vi "AlliGator Phasor Plot Image ROI Storage [MULT] v3.vi"(7 "Curent ROI Colors":u32[](array[colorbox]), 8 "Error In":errorcluster, 9 "Current ROI Descriptor(s)":T2[](array[typedef]) {"Contours"."Type" items=["No Selection", "Point", "Line", "Rectangle", "Oval", "Polygon", "Freehand Region", "Annulus", "Unused2", "Unused3", "Broken Line", "Freehand Line", "Rotated Rectangle"]}, 10 "Default Name(s) (\"ROI\")":string[](array[string]), 11 "Action":T1=enum."Update Current ROI Descriptor") -> (0 "Error Out":errorcluster, 1 "Current ROI Descriptors":T2[](array[typedef]) {"Contours"."Type" items=["No Selection", "Point", "Line", "Rectangle", "Oval", "Polygon", "Freehand Region", "Annulus", "Unused2", "Unused3", "Broken Line", "Freehand Line", "Rotated Rectangle"]}, 2 "Current ROI Names":string[](array[string]), 3 "Current Phasor Plot Image ROI":i32, 4 "Old ROI Name":string, 5 "Curent ROI Colors":u32[](array[colorbox]))   [LabVIEW 2021, in "AlliGator ROIs.lvlib"]
doc: "Handles multiple Phasor Plot image ROIs storage."
uses:
  AlliGator ROIs.lvlib
  AlliGator ROI Manager Actions.ctl
  Globals, Variables, Constants/AlliGator Variables List.ctl
  Image/Named ROI Description.ctl
  AlliGator Image ROI Event refnum.ctl
  Variant/Variant to Data/Variant to I32.vi
  <userlib>/_OpenG.lib/array/array.llb/Sort 1D Array (I32)__ogtk.vi
  Image/Image.lvlib
  Globals, Variables, Constants/AlliGator Globals, Variables & Constants.lvlib
  Variant/Variant to Data/Variant to Data.lvlib
  <userlib>/_OpenG.lib/array/array.llb/openg_array.lvlib
  Strings/Strings.lvlib
panel:
  # "see the AlliGator License on the block diagram (Ctrl+E or Window:Show Block Diagram)"
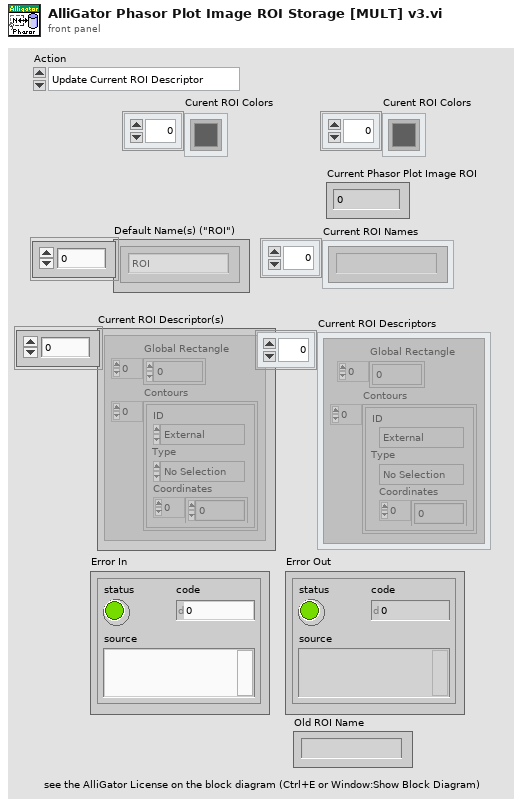
[diagram p1: front panel]
types:
  T1 = typedef "AlliGator ROIs.lvlib/AlliGator ROI Manager Actions.ctl" = enum16{"Undefined", "Delete Current ROI", "Delete All Unselected ROIs", "Delete Multiple ROIs", "Delete All ROIs", "Swap ROIs", "Insert ROI", "Update Current ROI Descriptor", "Rename Current ROI", "Store New ROI", "Store Multiple ROIs", "Select Next ROI", "Select Previous ROI", "Find Selected ROI", "Show All ROIs", "Update ROI Manager Window", "Merge All ROIs", "Unmerge ROI", "Set Selected ROI by ID"}
  T2 = typedef "ROI Descriptor" = cluster{"Global Rectangle":i32[], "Contours":cluster{"ID":enum32{"External", "Internal"}, "Type":u32, "Coordinates":i32[]}[]}
  T3 = typedef "AlliGator ROIs.lvlib/AlliGator Image ROI Event refnum.ctl" = refnum<user-event>
  T4 = typedef "AlliGator Globals, Variables & Constants.lvlib/AlliGator Variables List.ctl" = enum16{"---- GUI ----", "GUI:Initialization Status", "GUI:State Indicators Refnum", "GUI:Original AlliGator Menu Items", "GUI:Current Action Loop State", "GUI:Script in progress", "GUI:Playback", "GUI:Loop Playback", "GUI:Search ROI Used", "GUI:Search ROI", "Decay Graph Max Legend Size", "Intensity Graph Max Legend Size", "Decay Statistics Graph Max Legend Size", "Phasor Graph Max Legend Size", "Phasor Ratio Graph Max Legend Size", "Lifetime Graph Max Legend Size", "---- Files ----", "Files:Export Dataset Frames as Individual Files", "Files:Show Batch Export Help Balloons", "Files:Frames in Dataset", "Files:ptu File Frame Start Indices", "Files:Current Frame in Dataset", "Files:Current Frame Timestamp", "Files:Dataset Loaded", "Files:Dataset Metadata", "Files:Dataset Channel", "Files:Dataset Data Description", "Files:Background Dataset Metadata", "Files:Background Dataset Channel", "Files:Background Dataset Data Description", "Files:Background File Subtraction", "Files:Background File Path", "Files:Background File Pile-up Correction", "Files:Background File Pixel Well Capacity", "Files:Background File Scaling Factor", "Files:Current Dataset Load Settings", "Files:Dataset Path", "Files:ICCD-specific Information", "Files:Macrotime Gate Separation", "------ Python Plugins ------", "Python Plugins:Information", "Python Plugins:Python Session", "Python Plugins:Valid Python Session?", "---- Source Image ----", "Source Image:ROIs", "Source Image:Current ROI", "Source Image:ROI Event Refnum", "X_Source Image Display Range", "X_Source Image Palette Information", "X_Type of Displayed Image", "X_Time Gate Slider", "Source Image:Palette List", "Source Image:Scale", "Source Image:ROI Overlay Color", "Source Image:Overlay to Erase", "Source Image:Is Displayed Image Accumulated", "Source Image:White Light Image Modified", "Source Image:Mask Image Modified", "---- Image Profile Window ----", "Image Profile:Window Event Refnum", "Image Profile:IntensityType", "Image Profile:Intensity Average Type", "Image Profile:Intensity-weighted SDV", "Image Profile:Box Profile Type", "Image Profile:Window Open", "Image Profile:Plotted Fit Parameter", "------ Phasor Graph -------", "Phasor Graph:Show Line", "---- Phasor Plot ---", "Phasor Plot:Parameters Changed", "Phasor Plot:FLI Dataset Modified since last Calculation", "Phasor Harmonics Data", "Selected Phasor Harmonics", "Phasor Harmonic Manager Event Refnum", "Phasor Plot:ROIs", "Phasor Plot:Current ROI", "Phasor Plot:ROI Event Refnum", "Phasor Plot:Image Reference Points", "Phasor Plot:Computed", "Phasor Plot:Palette Information", "Phasor Plot:Palette List", "Phasor Plot:Phasor Ratio Palette Information", "Phasor Plot:Phasor Ratio Palette List", "Phasor Plot:Image Scale", "Phasor Plot:Image Overlay to Erase", "Phasor Plot:Image Elements to Update", "Phasor Plot:Current Calculation Parameters", "Phasor Plot:Current Calibration Options", "Phasor Plot:Reset Cumulated Phasor Plot", "Phasor Plot:Reference 1", "Phasor Plot:Lifetime Reference 1", "Phasor Plot:Reference 1 Frequency", "Phasor Plot:Reference 2", "Phasor Plot:Lifetime Reference 2", "Phasor Plot:Reference 2 Frequency", "---- Decay Analysis ----", "Number of Selected Decays to Fit", "LS Fit Results", "LAR Fit Results", "BS Fit Results", "Last Decay Max - Min", "Best Fit Parameters", "Best Fit Parameter Names", "Actual Size X", "Actual Size Y", "Binning X", "Binning Y", "Actual # Gates", "Dataset Number", "Gates to...", "Gates Skipped", "Gates to keep", "Gate Step", "Gate Separation", "Reversed Gates", "Pile-up Correction", "Pixel Well Capacity", "Background Subtracted", "Background Subtraction Method", "Background Definition Range", "Background File (deprecated)", "Number of Dataset Accumulated", "Array of Accumulated Dataset Paths", "Do Averaged Datasets", "Destination File Path", "Process Plot Target", "Use 1/D as Phasor Frequency", "---- Decay Fit Parameter Map -----", "Decay Fit Parameter Map:Palette Information", "Decay Fit Parameter Map:Palette List", "---- Parameter Map ----", "Parameter Map:Palette Information", "Parameter Map:Palette List", "------- Local Decay Window ---------", "Local Decay Graph Window:Event Refnum", "Local Decay Graph Window:Use normalized IRF for convolution", "----- Miscellaneous ----", "Misc:Skippable Dialog Windows Status"}
  T5 = typedef "Image.lvlib/Named ROI Description.ctl" = cluster{"ROI Descriptor":T2, "ROI Name":string, "Overlay Color":u32}
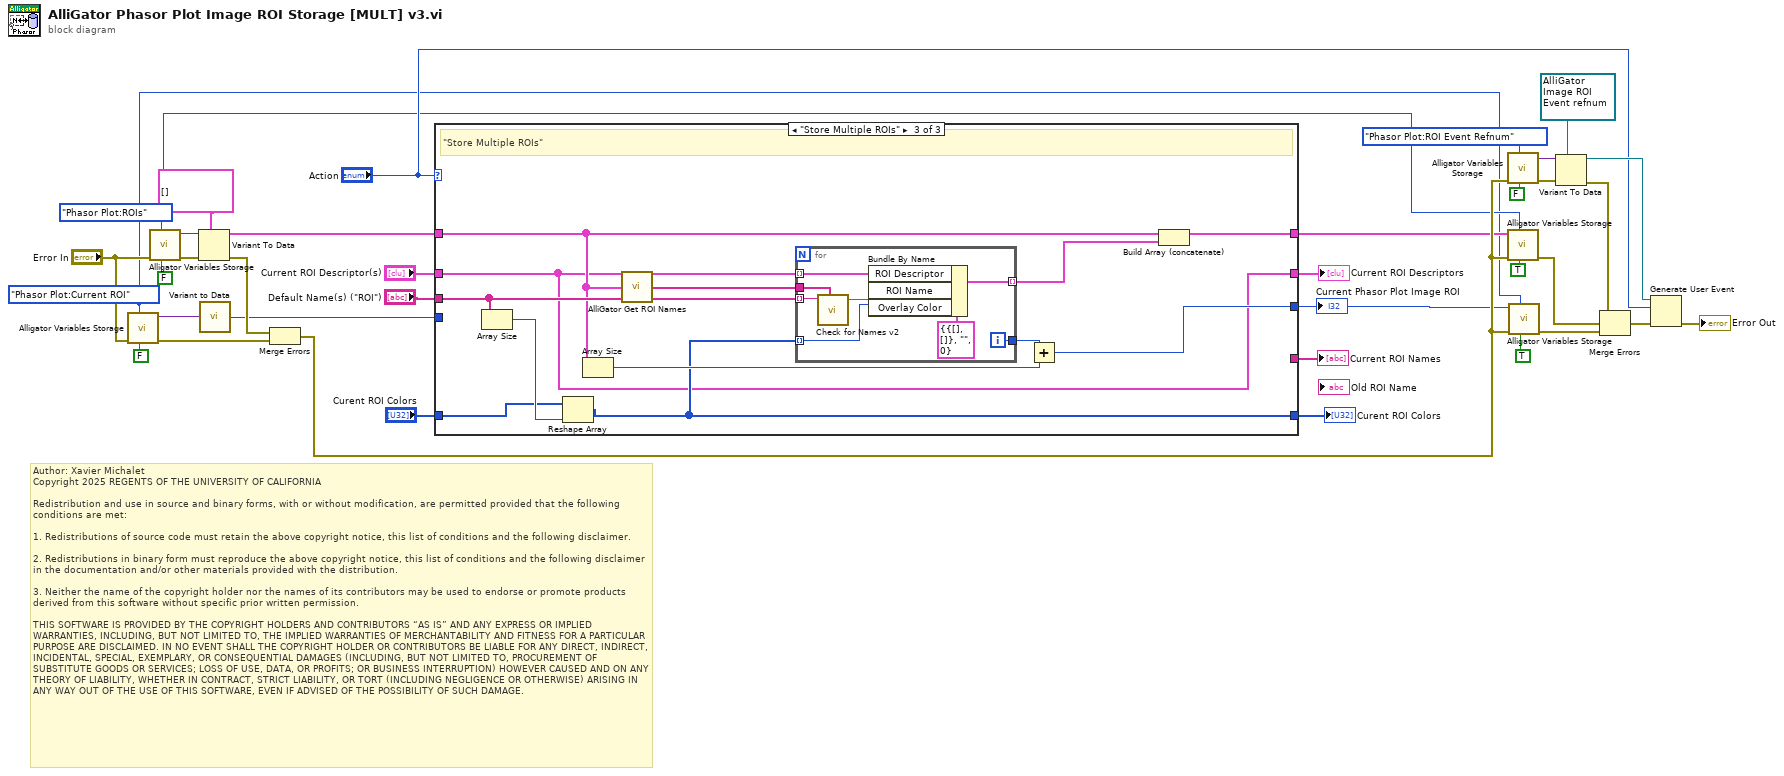
[diagram p0: block diagram]
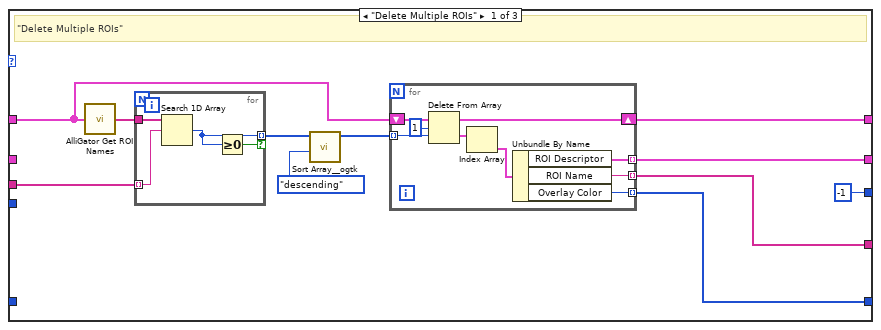
[diagram p2: hidden frame]
diagram:
  w16 = T3 refnum items=["Undefined", "Delete Current ROI", "Delete All Unselected ROIs", "Delete Multiple ROIs", "Delete All ROIs", "Swap ROIs", "Insert ROI", "Update Current ROI Descriptor", "Rename Current ROI", "Store New ROI", "Store Multiple ROIs", "Select Next ROI", "Select Previous ROI", "Find Selected ROI", "Show All ROIs", "Update ROI Manager Window", "Merge All ROIs", "Unmerge ROI", "Set Selected ROI by ID"] ("Source Image ROI Event Refnum")
  w1 = AlliGator_Variables_List."Phasor Plot:Current ROI" ("Alligator Variable")
  w2 = AlliGator_Variables_List."Phasor Plot:ROIs" ("Alligator Variable")
  # "Author: Xavier Michalet\nCopyright 2025 REGENTS OF THE UNIVERSITY OF CALIFORNIA\n\nRedistribution and use in source and binary forms, with or without modification, are permitted provided that the following conditions are met:\n\n1. Redistributions of source code must retain the above copyright notice, this list of conditions and the following disclaimer.\n\n2. Redistributions in binary form must reproduce the above copyright notice, this list of conditions and the following disclaimer in the documentation and/or other materials provided with the distribution.\n\n3. Neither the name of the copyright holder nor the names of its contributors may be used to endorse or promote products derived from this software without specific prior written permission.\n\nTHIS SOFTWARE IS PROVIDED BY THE COPYRIGHT HOLDERS AND CONTRIBUTORS “AS IS” AND ANY EXPRESS OR IMPLIED WARRANTIES, INCLUDING, BUT NOT LIMITED TO, THE IMPLIED WARRANTIES OF MERCHANTABILITY AND FITNESS FOR A PARTICULAR PURPOSE ARE DISCLAIMED. IN NO EVENT SHALL THE COPYRIGHT HOLDER OR CONTRIBUTORS BE LIABLE FOR ANY DIRECT, INDIRECT, INCIDENTAL, SPECIAL, EXEMPLARY, OR CONSEQUENTIAL DAMAGES (INCLUDING, BUT NOT LIMITED TO, PROCUREMENT OF SUBSTITUTE GOODS OR SERVICES; LOSS OF USE, DATA, OR PROFITS; OR BUSINESS INTERRUPTION) HOWEVER CAUSED AND ON ANY THEORY OF LIABILITY, WHETHER IN CONTRACT, STRICT LIABILITY, OR TORT (INCLUDING NEGLIGENCE OR OTHERWISE) ARISING IN ANY WAY OUT OF THE USE OF THIS SOFTWARE, EVEN IF ADVISED OF THE POSSIBILITY OF SUCH DAMAGE."
  n1 = call "Alligator Variables Storage.vi"("Get(F)/Set"=FALSE, "AlliGator Variable"=w1, "Error In"="Error In") -> ("Error Out"=w27:errorcluster, "Data out"=w31:variant)  [unwired: 6 in, 1 out]
  n2 = call "Alligator Variables Storage.vi"("Get(F)/Set"=FALSE, "AlliGator Variable"=w2, "Error In"="Error In") -> ("Error Out"=w35:errorcluster, "Data out"=w36:variant)  [unwired: 6 in, 1 out]
  n3 = Variant To Data(error in=w35, type=T5[] [] ("Stored ROIs in"), Variant=w36) -> (data=w13:T5[], error out=w26:errorcluster)
  n4 = call-poly "Variant to Data.vi"("Variant"=w31) -> ("Value"=w12:i32)  [unwired: 8 in]
  n5 = Merge Errors(w26, w27) -> (w19:errorcluster)
  n6 = case shown="\"Store Multiple ROIs\"" "Action" {
    tunnel: w13 -> [w41 w64 w70]
    tunnel: w12 -> [_ w62 _]
    tunnel: [w40 w64 w76] -> w9
    tunnel: [-1 ("Current ROI out") w62 w67] -> w8
    tunnel: "Current ROI Descriptor(s)" -> [_ w63 w65]
    tunnel: [w39 w63 w65] -> w7
    tunnel: "Default Name(s) (\"ROI\")" -> [w45 _ w73]
    tunnel: [w38 _ _] -> w6
    tunnel: [w37 w61 w66] -> w5
    tunnel: "Curent ROI Colors" -> [_ w61 w71]
    frame "Delete Multiple ROIs" {
      # "\"Delete Multiple ROIs\""
      n7 = call "AlliGator Get ROI Names.vi"("Stored ROIs in"=w41) -> ("ROI Name"=w46:string[])  [unwired: 8 in]
      n8 = for {
        tunnel: w46 -> [w60]
        tunnel: w45 -> [w59] mode=indexing
        tunnel: [w58] -> w44 mode=indexing if=w57
        n9 = Search 1D Array(1D array=w60, element=w59) -> (index of element=w58:i32)  [unwired: 1 in]
        n10 = Greater Or Equal To 0?(x=w58) -> (x >= 0?=w57:bool)
      }
      n11 = call-poly <userlib>:"Sort Array__ogtk.vi"("Order"=enum16{"ascending", "descending"}."descending", "Array in"=w44) -> ("Sorted Array out"=w42:i32[])  [unwired: 8 in, 1 out]
      n12 = for {
        tunnel: w42 -> [w56] mode=indexing
        shift-right: [w53] -> w40
        shift-left: w41 -> [w54]
        tunnel: [w50] -> w39 mode=indexing
        tunnel: [w49] -> w38 mode=indexing
        tunnel: [w48] -> w37 mode=indexing
        n13 = Delete From Array(array=w54, length=1, index=w56) -> (deleted portion=w52:T5[], array with subset deleted=w53:T5[])
        n14 = Index Array(array=w52) -> (element=w51:T5)  [unwired: 1 in]
        n15 = Unbundle By Name(w51) -> ("ROI Descriptor"=w50:T2, "ROI Name"=w49:string, "Overlay Color"=w48:u32)
      }
    }
    frame Default {
      # "Default"
    }
    frame "Store Multiple ROIs" {
      # "\"Store Multiple ROIs\""
      n16 = Array Size(array=w73) -> (size(s)=w72:i32)
      n17 = Reshape Array(w71, w72) -> (w66:u32[])
      n18 = Array Size(array=w70) -> (size(s)=w68:i32)
      n19 = call "AlliGator Get ROI Names.vi"("Stored ROIs in"=w70) -> ("ROI Name"=w74:string[])  [unwired: 8 in]
      n20 = for {
        tunnel: w65 -> [w82] mode=indexing
        tunnel: [w83] -> w75 mode=indexing
        tunnel: w73 -> [w80] mode=indexing
        tunnel: w74 -> [w81]
        tunnel: [w78] -> w69
        tunnel: w66 -> [w77] mode=indexing
        i -> [w78]
        n21 = call "Check for Names v2.vi"("New Name"=w80, "Name List"=w81) -> ("New Name"=w79:string)  [unwired: 4 in, 3 out]
        n22 = Bundle By Name(cluster=T5 {"ROI Descriptor"={"Global Rectangle"=[], "Contours"=[]}, "ROI Name"="", "Overlay Color"=0} ("Named ROI Description"), "ROI Descriptor"=w82, "ROI Name"=w79, "Overlay Color"=w77) -> (w83:T5)
      }
      n23 = Add(x=w69, y=w68) -> (x+y=w67:i32)
      n24 = Build Array (concatenate)(w70, w75) -> (w76:T5[])
    }
  }
  "Current ROI Descriptors" <- w7
  "Current Phasor Plot Image ROI" <- w8
  "Current ROI Names" <- w6
  "Curent ROI Colors" <- w5
  n25 = call "Alligator Variables Storage.vi"("Get(F)/Set"=FALSE, "AlliGator Variable"=AlliGator_Variables_List."Phasor Plot:ROI Event Refnum" ("Alligator Variable"), "Error In"=w19) -> ("Error Out"=w18:errorcluster, "Data out"=w17:variant)  [unwired: 6 in, 1 out]
  n26 = call "Alligator Variables Storage.vi"("Get(F)/Set"=TRUE, "AlliGator Variable"=w2, "Error In"=w19, "Data in"=w9) -> ("Error Out"=w24:errorcluster)  [unwired: 5 in, 2 out]
  n27 = call "Alligator Variables Storage.vi"("Get(F)/Set"=TRUE, "AlliGator Variable"=w1, "Error In"=w19, "Data in"=w8) -> ("Error Out"=w25:errorcluster)  [unwired: 5 in, 2 out]
  n28 = Variant To Data(error in=w18, type=w16, Variant=w17) -> (data=w15:T3, error out=w14:errorcluster)
  n29 = Merge Errors(w14, w24, w25) -> (w23:errorcluster)
  n30 = Generate User Event(user event=w15, event data cluster="Action", error in=w23) -> (error out=→"Error Out":errorcluster)  [unwired: 1 in, 1 out]
